vi "KundtsTube.vi"() -> ()   [LabVIEW 2015]
panel:
  in  "# of Samples":i32
  in  "Sampling Rate (Hz)":dbl
  out "Waveform":dynamicdata(graph)
  out "Gain vs Freq":cluster{i32[], dbl[]}(graph)
  in  "stop":bool
  in  "Amplitude":dbl
  in  "Tab Control":enum32{"Sweep", "Single"}(tab)
  in  "Dwell Time, sec":dbl format="%#_6f"
  in  "Frequency":dbl format="%.1f"
  out "Output":cluster{"rms value":dbl, "Frequency":i32} {"rms value" format="%0.2f"}
  in  "Int Array Control":T1={"Minimum"=10, "Maximum"=10000, "# of Points"=1999, "Spacing"=enum."Linear"}
  # "Sweeps through frequencies defined\nat right, pausing between for below\ndwell time"
  # "Runs at below defined frequency"
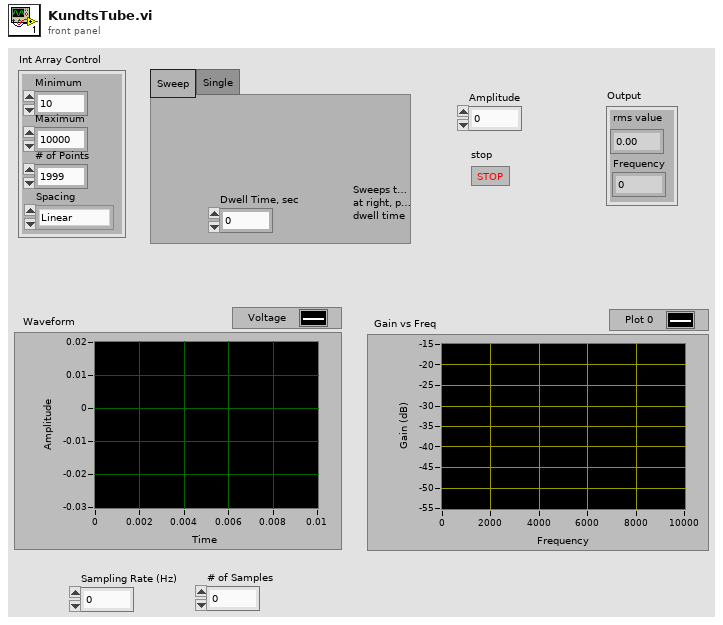
[diagram p1: front panel]
types:
  T1 = cluster{"Minimum":i32, "Maximum":i32, "# of Points":i32, "Spacing":enum16{"Linear", "Logarithmic"}}
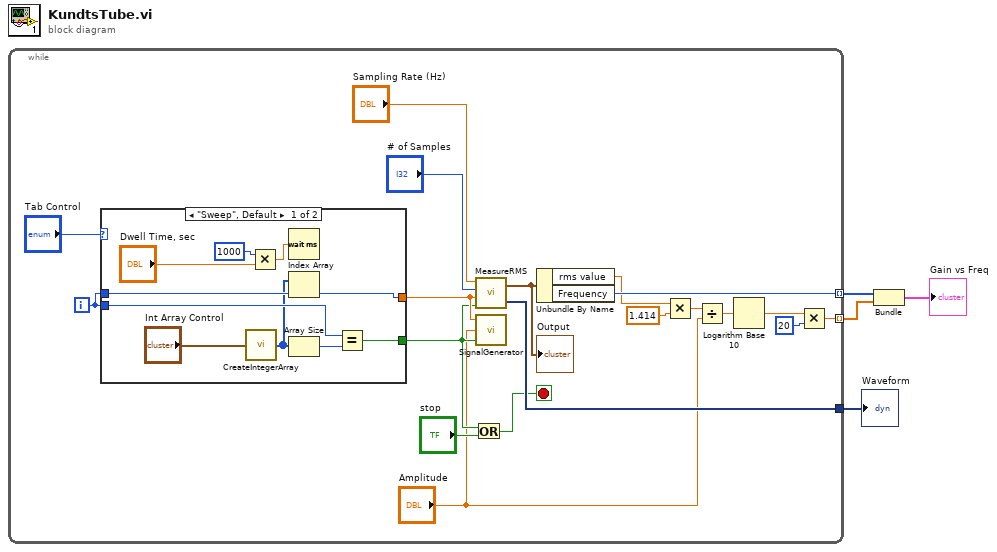
[diagram p0: block diagram]
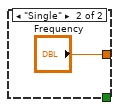
[diagram p2: hidden frame]
diagram:
  n1 = while {
    tunnel: [w16] -> w4 mode=indexing
    tunnel: [w15] -> w3 mode=indexing
    tunnel: [w14] -> w1
    i -> [w12]
    stop <- w10 stop-if-true
    n2 = case shown="\"Sweep\", Default" "Tab Control" {
      tunnel: w12 -> [w29 _]
      tunnel: [w28 "Frequency"] -> w17
      tunnel: w12 -> [w26 _]
      tunnel: [w24 _] -> w9
      frame "Sweep", Default {
        n3 = call "CreateIntegerArray.vi"("Int Array"="Int Array Control") -> ("Array"=w25:i32[])
        n4 = Multiply(x=1000, y="Dwell Time, sec") -> (x*y=w33:dbl)
        n5 = Wait (ms)(milliseconds to wait=w33) -> ()  [unwired: 1 out]
        n6 = Index Array(array=w25, index=w29) -> (element=w28:i32)
        n7 = Array Size(array=w25) -> (size(s)=w27:i32)
        n8 = Equal?(x=w26, y=w27) -> (x = y?=w24:bool)
      }
      frame "Single" {
      }
    }
    n9 = Or(x=w9, y="stop") -> (x .or. y?=w10:bool)
    n10 = call "MeasureRMS.vi"("stop (T)"=w9, "Frequency"=w17, "# of Samples"="# of Samples", "Sampling Rate (Hz)"="Sampling Rate (Hz)") -> ("Waveform Graph"=w14:dynamicdata, "Output"=w13:cluster{"rms value":dbl, "Frequency":i32})
    "Output" <- w13
    n11 = call "SignalGenerator.vi"("stop"=w9, "Amplitude"="Amplitude", "Frequency"=w17) -> ()  [unwired: 1 in]
    n12 = Unbundle By Name(w13) -> ("rms value"=w7:dbl, "Frequency"=w16:i32)
    n13 = Multiply(x=w7, y=1.414) -> (x*y=w6:dbl)
    n14 = Divide(x=w6, y="Amplitude") -> (x/y=w20:dbl)
    n15 = Logarithm Base 10(1:w20) -> (0:w21:dbl)
    n16 = Multiply(x=w21, y=20) -> (x*y=w15:dbl)
  }
  "Waveform" <- w1
  n17 = Bundle(w4, w3) -> (→"Gain vs Freq":cluster{i32[], dbl[]})  [unwired: 1 in]
